vi "CA Spec.vi"(3 "df":dbl, 4 "FFT size":u16, 5 "Array":dbl[](array[numeric])) -> (1 "f diff":dbl, 2 "Spectro fig":dbl[][](graph))   [LabVIEW 2022 SP3]
uses:
  <vilib>/Analysis/baseanly.llb/Mean (DBL).vi
  <vilib>/gmath/NI_Gmath.lvlib
  <vilib>/Analysis/NI_AALBase.lvlib
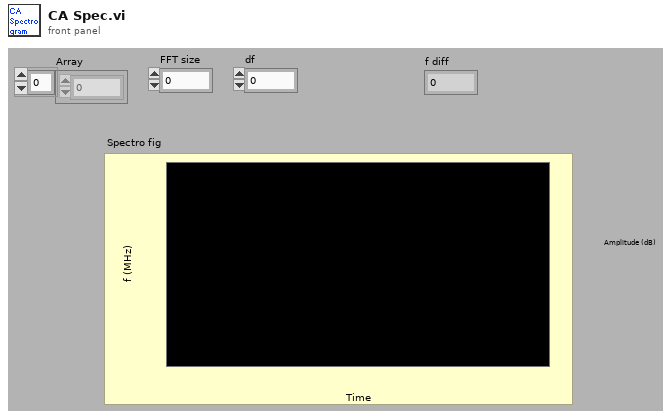
[diagram p1: front panel]
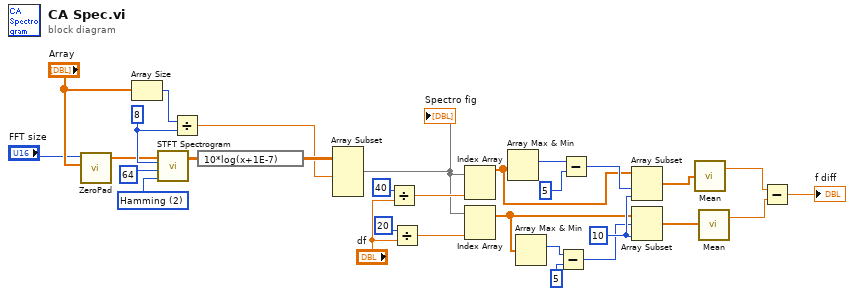
[diagram p0: block diagram]
diagram:
  w12 = 2 items=["Rectangular", "Blackman", "Hamming", "Hanning", "Gaussian"] ("window selector")
  w21 = 8 ("time increment")
  w26 = 10
  n1 = call "ZeroPad.vi"("Input Array"="Array", "FFT size"="FFT size") -> ("Ouput Array"=w14:dbl[])  [unwired: 4 out]
  n2 = Array Size(array="Array") -> (size(s)=w19:i32)
  n3 = call <vilib>:"STFT Spectrogram.vi"("window selector"=w12, "window length"=64 ("window pts"), "time increment"=w21, "X"=w14) -> ("STFT Spectrogram {X}"=w22:dbl[][])  [unwired: 1 out]
  n4 = Divide(x=w19, y=w21) -> (x/y=w9:dbl)
  n5 = expression code="10*log(x+1E-7)"(w22) -> (w11:dbl[][])
  n6 = Array Subset(array=w11, length (row)=w9) -> (w10:dbl[][])  [unwired: 3 in]
  "Spectro fig" <- w10
  n7 = Divide(x=40, y="df") -> (x/y=w16:dbl)
  n8 = Divide(x=20, y="df") -> (x/y=w15:dbl)
  n9 = Index Array(array=w10, index (col)=w16) -> (element=w7:dbl[])  [unwired: 1 in]
  n10 = Index Array(array=w10, index (col)=w15) -> (element=w6:dbl[])  [unwired: 1 in]
  n11 = Array Max & Min(array=w7) -> (max index (indices)=w24:i32)  [unwired: 3 out]
  n12 = Array Max & Min(array=w6) -> (max index (indices)=w5:i32)  [unwired: 3 out]
  n13 = Subtract(x=w5, y=5) -> (x-y=w4:i32)
  n14 = Subtract(x=w24, y=5) -> (x-y=w8:i32)
  n15 = Array Subset(array=w7, index=w8, length=w26) -> (w2:dbl[])
  n16 = Array Subset(array=w6, index=w4, length=w26) -> (w3:dbl[])
  n17 = call-poly <vilib>:"Mean.vi"("X"=w2) -> ("mean"=w27:dbl)  [unwired: 1 out]
  n18 = call-poly <vilib>:"Mean.vi"("X"=w3) -> ("mean"=w28:dbl)  [unwired: 1 out]
  n19 = Subtract(x=w27, y=w28) -> (x-y=→"f diff":dbl)
